vi "VNA_Set_Trace_Number.vi"(2 "error in (no error)":errorcluster, 3 "Number of Traces":i32=1, 4 "VISA resource in":refnum<visa-resource-name>) -> (0 "error out":errorcluster, 1 "VISA VNA out":refnum<visa-resource-name>)   [LabVIEW 2017]
panel:
  in  "Active Channel":i32=1
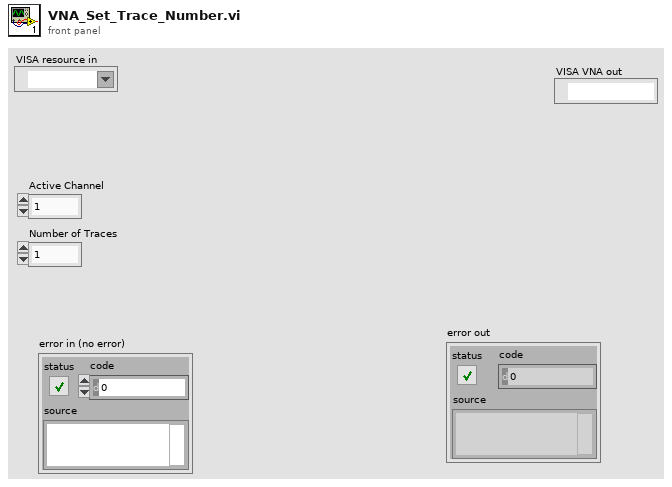
[diagram p1: front panel]
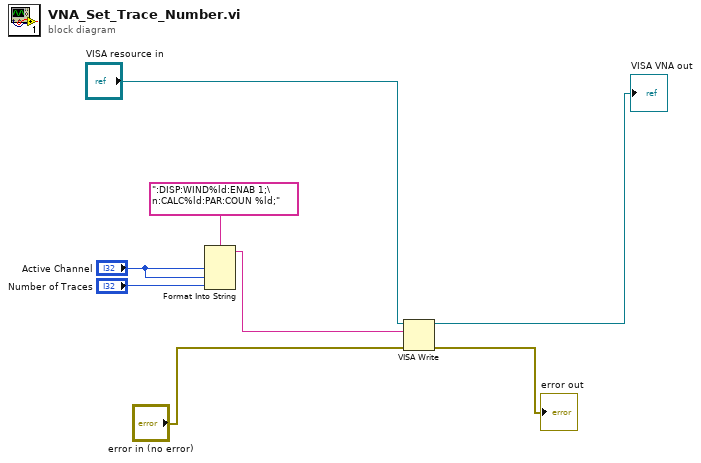
[diagram p0: block diagram]
diagram:
  n1 = Format Into String(format string=":DISP:WIND%ld:ENAB 1;\n:CALC%ld:PAR:COUN %ld;", "Active Channel", "Active Channel", "Number of Traces") -> (resulting string=w5:string)  [unwired: 2 in, 1 out]
  n2 = VISA Write(VISA resource name="VISA resource in", write buffer=w5, error in (no error)="error in (no error)") -> (VISA resource name out=→"VISA VNA out":refnum<visa-resource-name>, error out=→"error out":errorcluster)  [unwired: 1 out]
